vi "CoilsTest.vi"() -> ()   [LabVIEW 2012]
panel:
  out "error out":errorcluster
  in  "Coils":T1={"AO Channels"="DAC_COILS/ao0:3", "DO Lines"="DAC_COILS/port0/line0:1, DAC_COILS/port0/line8:9", "Settings"={"x"=0.0, "y"=0.0, "z"=0.0, "axgrad"=0.0}, "Keithley USB"="", "Current Toggle"=FALSE, "AO Task"="", "DO Task"=""}
  in  "Stop":bool
  # "(A)"
  # "(A)"
  # "(A)"
  # "(DAC V)"
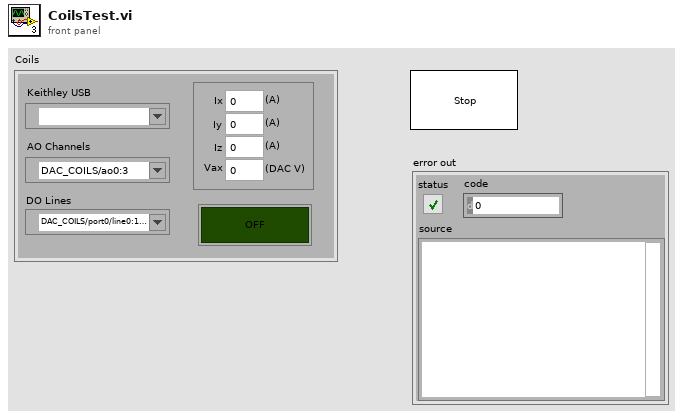
[diagram p1: front panel]
types:
  T1 = cluster{"AO Channels":tag, "DO Lines":tag, "Settings":cluster{"x":dbl, "y":dbl, "z":dbl, "axgrad":dbl}, "Keithley USB":refnum<visa-resource-name>, "Current Toggle":bool, "AO Task":refnum<k21>, "DO Task":refnum<k21>}
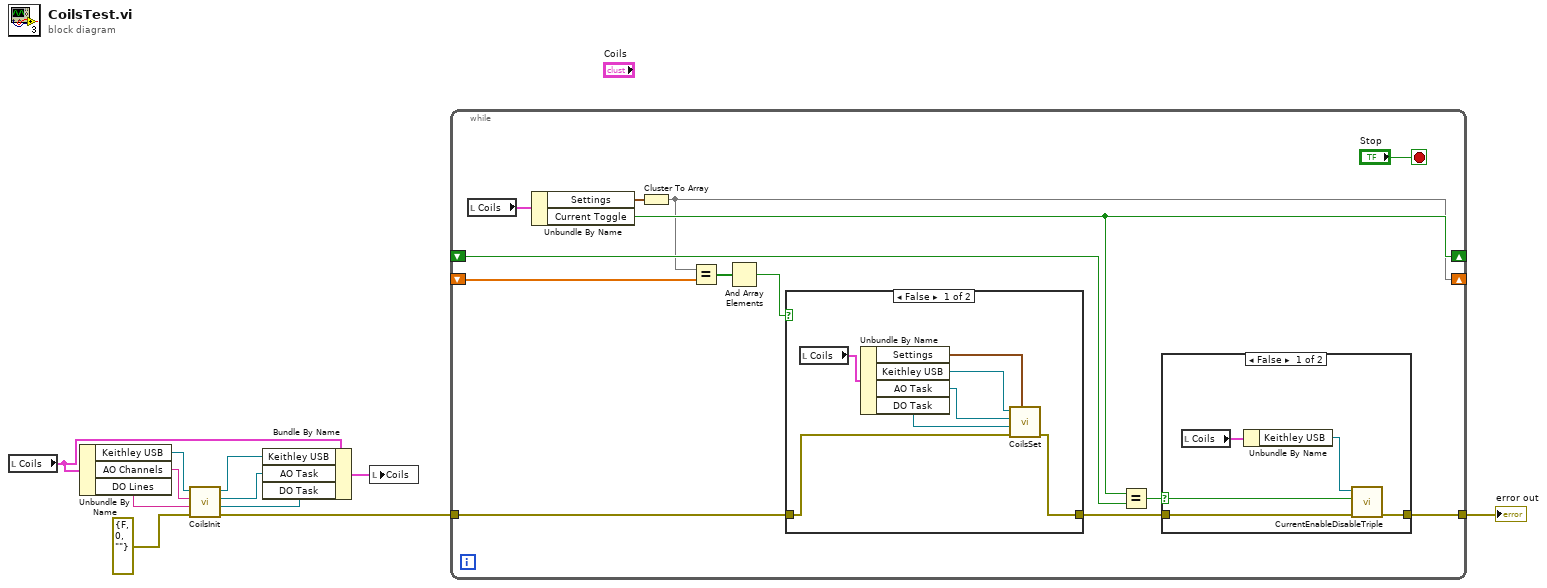
[diagram p0: block diagram]
diagram:
  n1 = local read "Coils"() -> (w5:T1)
  n2 = Unbundle By Name(w5) -> ("Keithley USB"=w8:refnum<visa-resource-name>, "AO Channels"=w7:tag, "DO Lines"=w6:tag)
  n3 = call "CoilsInit.vi"("error in"=errorcluster {"status"=FALSE, "code"=0, "source"=""}, "DO Lines"=w6, "AO Channels"=w7, "Keithley USB"=w8) -> ("error out"=w11:errorcluster, "DO Task out"=w1:refnum<k21>, "AO Task out"=w2:refnum<k21>, "Keithley USB out"=w3:refnum<visa-resource-name>)  [unwired: 4 in]
  n4 = Bundle By Name(cluster=w5, "Keithley USB"=w3, "AO Task"=w2, "DO Task"=w1) -> (w4:T1)
  n5 = local write "Coils"(w4) -> ()
  n6 = while {
    shift-right: [w22] -> _
    shift-left: _ -> [w21]
    shift-right: [w18] -> _
    shift-left: _ -> [w17]
    tunnel: w11 -> [w16]
    tunnel: [w14] -> w10
    stop <- "Stop" stop-if-true
    n7 = local read "Coils"() -> (w23:T1)
    n8 = Unbundle By Name(w23) -> ("Settings"=w19:cluster{"x":dbl, "y":dbl, "z":dbl, "axgrad":dbl}, "Current Toggle"=w22:bool)
    n9 = Cluster To Array(cluster=w19) -> (array=w18:dbl[])
    n10 = Equal?(x=w18, y=w17) -> (x = y?=w13:bool[])
    n11 = And Array Elements(Boolean array=w13) -> (logical AND=w12:bool)
    n12 = case shown="False" w12 {
      tunnel: w16 -> [w27 w32]
      tunnel: [w26 w32] -> w15
      frame False {
        n13 = local read "Coils"() -> (w25:T1)
        n14 = Unbundle By Name(w25) -> ("Settings"=w31:cluster{"x":dbl, "y":dbl, "z":dbl, "axgrad":dbl}, "Keithley USB"=w30:refnum<visa-resource-name>, "AO Task"=w29:refnum<k21>, "DO Task"=w28:refnum<k21>)
        n15 = call "CoilsSet.vi"("Settings"=w31, "error in"=w27, "DO Task"=w28, "AO Task"=w29, "Keithley USB"=w30) -> ("error out"=w26:errorcluster)  [unwired: 3 in, 3 out]
      }
      frame True {
      }
    }
    n16 = Equal?(x=w22, y=w21) -> (x = y?=w20:bool)
    n17 = case shown="False" w20 {
      selector: w20 -> [w33 _]
      tunnel: [w36 w38] -> w14
      tunnel: w15 -> [w37 w38]
      frame False {
        n18 = local read "Coils"() -> (w35:T1)
        n19 = Unbundle By Name(w35) -> ("Keithley USB"=w34:refnum<visa-resource-name>)
        n20 = call "CurrentEnableDisableTriple.vi"("error in (no error)"=w37, "Enable Output (T: On)"=w33, "Visa Resource Name In"=w34) -> ("error in (no error) 2"=w36:errorcluster)  [unwired: 7 in, 1 out]
      }
      frame True {
      }
    }
  }
  "error out" <- w10
